vi "CreatePublicEvents.vi"(8 "error in (no error)":errorcluster, 11 "RemoteControl":refnum<class "RemoteControl.lvclass">) -> (0 "error out":errorcluster, 3 "RemoteControl out":refnum<class "RemoteControl.lvclass">)   [LabVIEW 2019, in "RemoteControl.lvlib" / "RemoteControl.lvclass"]
doc: "---------------------------------------------------------------\nJKI State Machine Objects™\nhttp://jki.net/state-machine-objects/\nCopyright (C) 2005-2015, JKI <info@jki.net>\nALL RIGHTS RESERVEDJKI State Machine Objects (SMO) 1.0.0.4\nJKI - JKI\nCopyright (c) 2015, JKI"
uses:
  RemoteControl.lvclass
  Typedefs/PublicEvents--RemoteControl.SendMessageFromProcess.ctl
  Typedefs/Message--Cluster.ctl
  RemoteControl.lvclass/RemoteControl.ctl
  <vilib>/JKI/JKI SMO/smo.lvlibp/SMO/SMO.lvclass
panel:
  # "For instructions on how to use the JKI State Machine Objects, examples and video tutorials, visit:\nhttp://jki.net/state-machine-objects/\n\nJKI State Machine Objects™\nhttp://jki.net/state-machine-objects/\nCopyright (C) 2005-2015, JKI <info@jki.net>\nALL RIGHTS RESERVED"
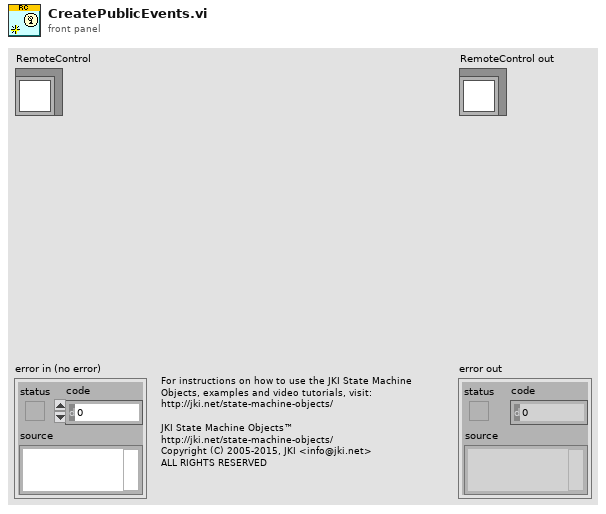
[diagram p1: front panel]
types:
  T1 = typedef "RemoteControl.lvlib/RemoteControl.lvclass/PublicEvents--RemoteControl.SendMessageFromProcess.ctl" = cluster{"Message":T2}
  T2 = typedef "RemoteControl.lvlib/RemoteControl.lvclass/Message--Cluster.ctl" = cluster{"Command":string, "Data":variant, "ID":string}
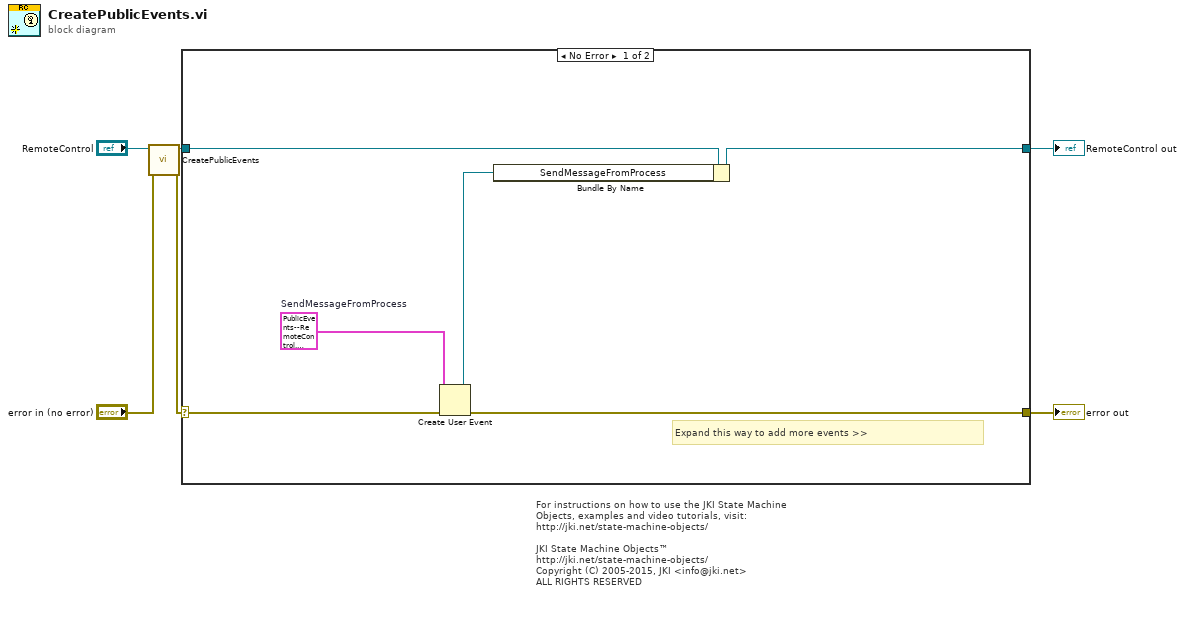
[diagram p0: block diagram]
diagram:
  # "For instructions on how to use the JKI State Machine Objects, examples and video tutorials, visit:\nhttp://jki.net/state-machine-objects/\n\nJKI State Machine Objects™\nhttp://jki.net/state-machine-objects/\nCopyright (C) 2005-2015, JKI <info@jki.net>\nALL RIGHTS RESERVED"
  n1 = call-parent "CreatePublicEvents.vi"("error in (no error)"="error in (no error)", "SMO"="RemoteControl") -> ("error out"=w1:errorcluster, "SMO out"=w3:refnum<class "RemoteControl.lvclass">)  [unwired: 8 in]
  n2 = case shown="No Error" w1 {
    selector: w1 -> [w7 w14]
    tunnel: [w10 w14] -> w5
    tunnel: [w11 w13] -> w6
    tunnel: w3 -> [w12 w13]
    frame No Error {
      w9 = T1 {"Message"={"Command"="", "Data"=variant(string ""), "ID"=""}}  # SendMessageFromProcess
      # "Expand this way to add more events >>"
      n3 = Create User Event(user event datatype=w9, error in=w7) -> (user event=w8:refnum<user-event>, error out=w10:errorcluster)
      n4 = Bundle By Name(cluster=w12, "SendMessageFromProcess"=w8) -> (w11:refnum<class "RemoteControl.lvclass">)
    }
    frame Error {
    }
  }
  "error out" <- w5
  "RemoteControl out" <- w6
